vi "Real SOL.vi"() -> ()   [LabVIEW 2016]
panel:
  in  "СТОП":bool
  in  "Solar 5":bool
  in  "Engine":bool
  in  "cubesat 3":bool
  in  "roboarm":bool
  # "REAL SOLUTIONS"
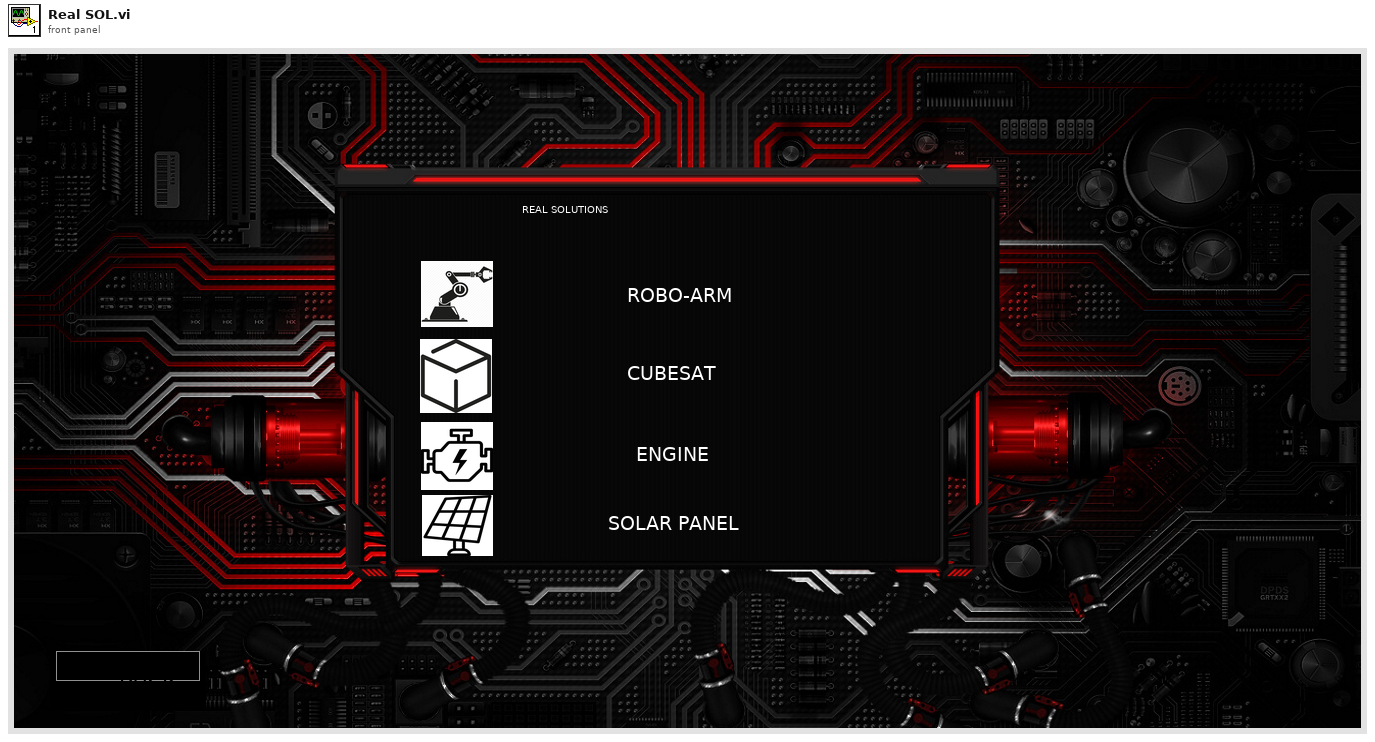
[diagram p1: front panel]
types:
  T1 = enum32{"Invalid", "Standard", "Closed", "Hidden", "Minimized", "Maximized"}
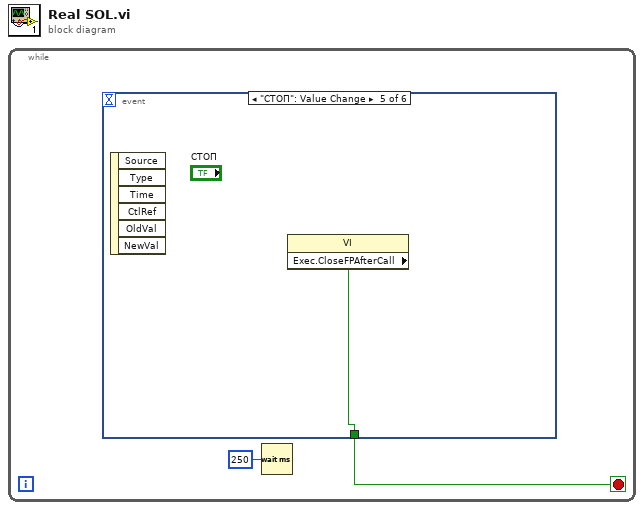
[diagram p0: block diagram]
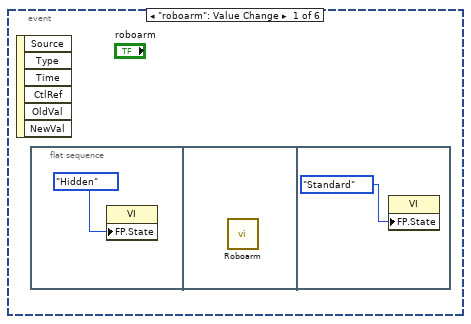
[diagram p2: hidden frame]
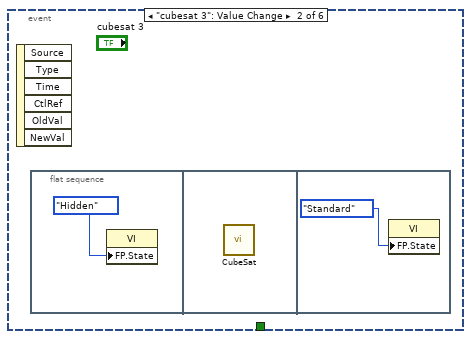
[diagram p3: hidden frame]
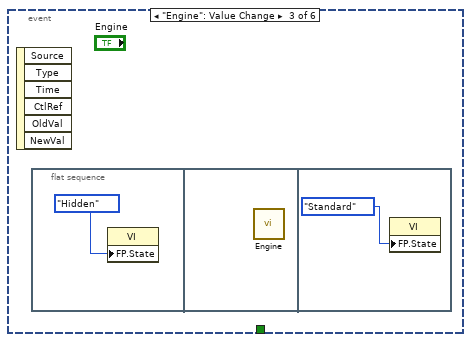
[diagram p4: hidden frame]
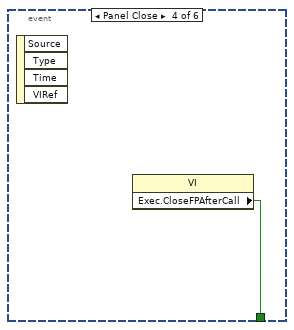
[diagram p5: hidden frame]
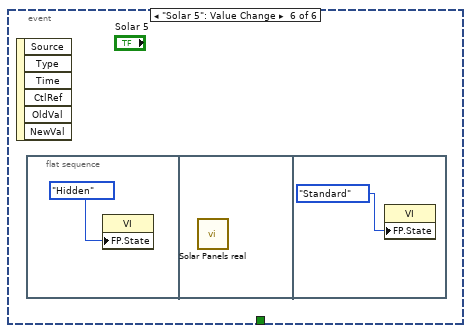
[diagram p6: hidden frame]
diagram:
  n1 = while {
    stop <- w1 stop-if-true
    n2 = event shown="[4] \"СТОП\": Value Change" {
      selector: _ -> [_ _ _ _ _ _]
      dyn-events: _ -> [_ _ _ _ _ _]
      timeout: _ -> [_ _ _ _ _ _]
      tunnel: [_ _ _ w9 w10 _] -> w1
      event "roboarm": Value Change {
        n3 = event-data() -> ()  [unwired: 1 in, 6 out]
        n4 = flat-sequence {
          frame #0 {
            n5 = property class="VI"("FP.State"=T1."Hidden" ("Front Panel Window:State")) -> ()  [unwired: 2 in, 2 out]
          }
          frame #1 {
            n6 = call "Roboarm.vi"() -> ()  [unwired: 12 in]
          }
          frame #2 {
            n7 = property class="VI"("FP.State"=T1."Standard" ("Front Panel Window:State")) -> ()  [unwired: 2 in, 2 out]
          }
        }
      }
      event "cubesat 3": Value Change {
        n8 = event-data() -> ()  [unwired: 1 in, 6 out]
        n9 = flat-sequence {
          frame #0 {
            n10 = property class="VI"("FP.State"=T1."Hidden" ("Front Panel Window:State")) -> ()  [unwired: 2 in, 2 out]
          }
          frame #1 {
            n11 = call "CubeSat.vi"() -> ()  [unwired: 12 in]
          }
          frame #2 {
            n12 = property class="VI"("FP.State"=T1."Standard" ("Front Panel Window:State")) -> ()  [unwired: 2 in, 2 out]
          }
        }
      }
      event "Engine": Value Change {
        n13 = event-data() -> ()  [unwired: 1 in, 6 out]
        n14 = flat-sequence {
          frame #0 {
            n15 = property class="VI"("FP.State"=T1."Hidden" ("Front Panel Window:State")) -> ()  [unwired: 2 in, 2 out]
          }
          frame #1 {
            n16 = call "Engine.vi"() -> ()  [unwired: 12 in]
          }
          frame #2 {
            n17 = property class="VI"("FP.State"=T1."Standard" ("Front Panel Window:State")) -> ()  [unwired: 2 in, 2 out]
          }
        }
      }
      event Panel Close {
        n18 = event-data() -> ()  [unwired: 1 in, 4 out]
        n19 = property class="VI"() -> ("Exec.CloseFPAfterCall"=w9:bool)  [unwired: 2 in, 2 out]
      }
      event "СТОП": Value Change {
        n20 = event-data() -> ()  [unwired: 1 in, 6 out]
        n21 = property class="VI"() -> ("Exec.CloseFPAfterCall"=w10:bool)  [unwired: 2 in, 2 out]
      }
      event "Solar 5": Value Change {
        n22 = event-data() -> ()  [unwired: 1 in, 6 out]
        n23 = flat-sequence {
          frame #0 {
            n24 = property class="VI"("FP.State"=T1."Hidden" ("Front Panel Window:State")) -> ()  [unwired: 2 in, 2 out]
          }
          frame #1 {
            n25 = call "Solar Panels real.vi"() -> ()  [unwired: 12 in]
          }
          frame #2 {
            n26 = property class="VI"("FP.State"=T1."Standard" ("Front Panel Window:State")) -> ()  [unwired: 2 in, 2 out]
          }
        }
      }
    }
    n27 = Wait (ms)(milliseconds to wait=u32 250) -> ()  [unwired: 1 out]
  }
